vi "PQfetchResultData_experiment.vi"() -> ()   [LabVIEW 2019, in "libpqutility.lvlib"]
uses:
  libpqutility.lvlib
  libpqlv/libpqlv.lvlib
panel:
  in  "conninfo":T1={"host"="localhost", "port"="5432", "client_encoding"="WIN1251", "dbname"="data", "user"="postgres", "password"=""}
  in  "Command":string
  out "DatabaseMesssageCluster":T2
  out "Data":string[][](table)
  out "error out":errorcluster
  in  "error in":errorcluster
  out "PQnTuples":u32
  out "PQnFields":u32
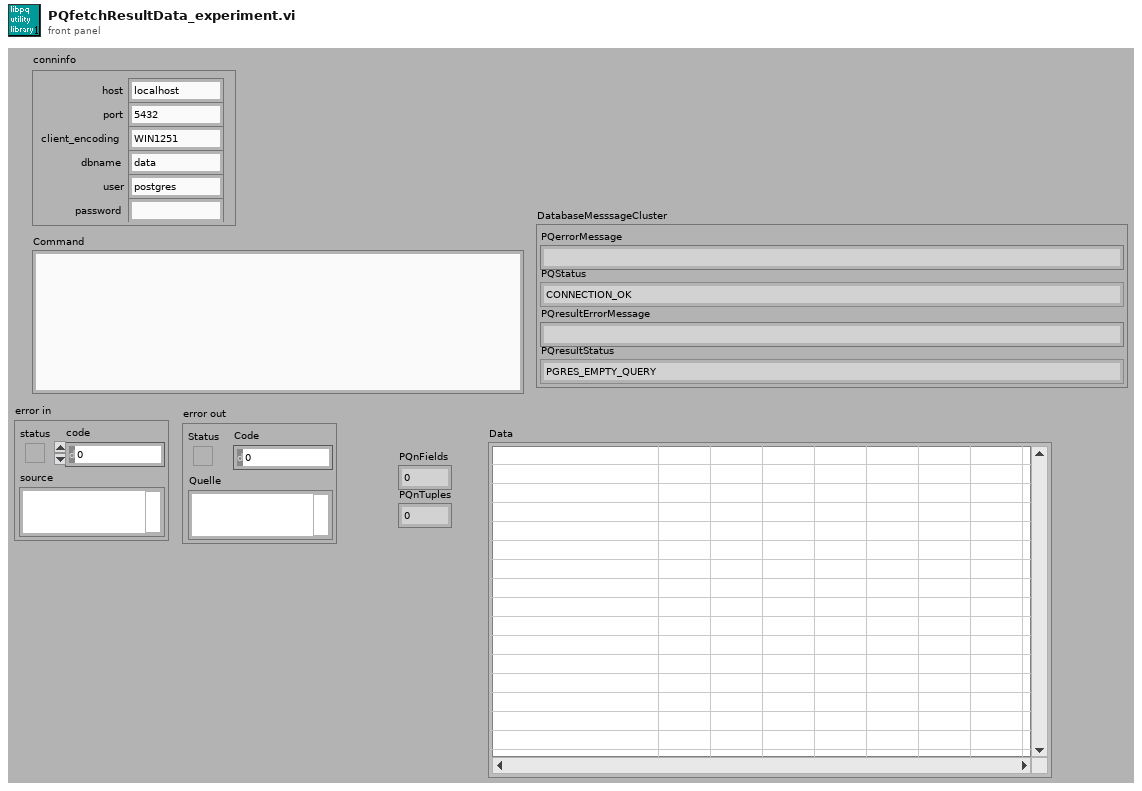
[diagram p1: front panel]
types:
  T1 = cluster{"host":string, "port":string, "client_encoding":string, "dbname":string, "user":string, "password":string}
  T2 = cluster{"PQerrorMessage":string, "PQStatus":enum16{"CONNECTION_OK", "CONNECTION_BAD", "CONNECTION_STARTED", "CONNECTION_MADE", "CONNECTION_AWAITING_RESPONSE", "CONNECTION_AUTH_OK", "CONNECTION_SETENV", "CONNECTION_SSL_STARTUP", "CONNECTION_NEEDED"}, "PQresultErrorMessage":string, "PQresultStatus":enum16{"PGRES_EMPTY_QUERY", "PGRES_COMMAND_OK", "PGRES_TUPLES_OK", "PGRES_COPY_OUT", "PGRES_COPY_IN", "PGRES_BAD_RESPONSE", "PGRES_NONFATAL_ERROR", "PGRES_FATAL_ERROR"}}
  T3 = enum32{"CONNECTION_OK", "CONNECTION_BAD", "CONNECTION_STARTED", "CONNECTION_MADE", "CONNECTION_AWAITING_RESPONSE", "CONNECTION_AUTH_OK", "CONNECTION_SETENV", "CONNECTION_SSL_STARTUP", "CONNECTION_NEEDED"}
  T4 = enum16{"PGRES_EMPTY_QUERY", "PGRES_COMMAND_OK", "PGRES_TUPLES_OK", "PGRES_COPY_OUT", "PGRES_COPY_IN", "PGRES_BAD_RESPONSE", "PGRES_NONFATAL_ERROR", "PGRES_FATAL_ERROR"}
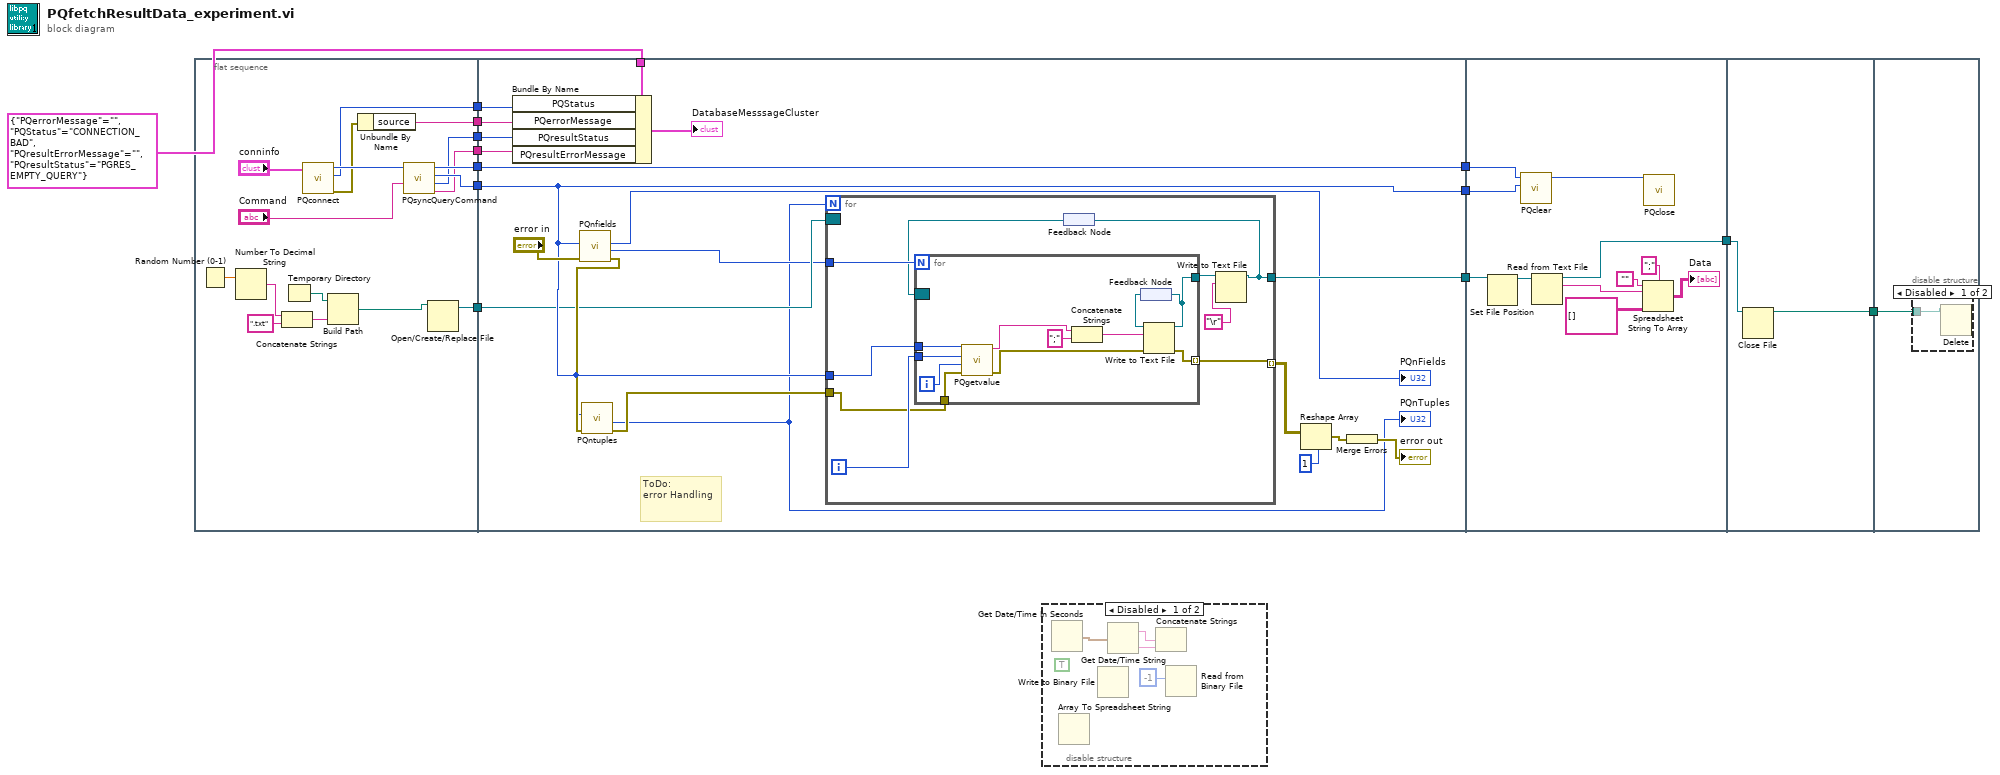
[diagram p0: block diagram]
diagram:
  n1 = flat-sequence {
    tunnel: [w27] -> w10
    tunnel: [w26] -> w8
    tunnel: [w16] -> w6
    tunnel: [w14] -> w5
    tunnel: [w25] -> w4
    tunnel: [w24] -> w3
    tunnel: [w19] -> w1
    tunnel: [w43] -> w13
    tunnel: [w42] -> w11
    tunnel: w10 -> [w42]
    tunnel: [w41] -> w9
    tunnel: w8 -> [w41]
    tunnel: T2 {"PQerrorMessage"="", "PQStatus"=enum."CONNECTION_BAD", "PQresultErrorMessage"="", "PQresultStatus"=enum."PGRES_EMPTY_QUERY"} ("Database Status Message 2") -> [w39]
    tunnel: w6 -> [w38]
    tunnel: w5 -> [w37]
    tunnel: w4 -> [w36]
    tunnel: w3 -> [w35]
    tunnel: w1 -> [w34]
    tunnel: w13 -> [w76]
    tunnel: [w80] -> w12
    tunnel: w11 -> [w78]
    tunnel: w9 -> [w77]
    tunnel: w12 -> [w83]
    tunnel: [w82] -> w2
    tunnel: w2 -> [w84]
    frame #0 {
      n2 = Random Number (0-1)() -> (number: 0 to 1=w29:dbl)
      n3 = Number To Decimal String(number=w29) -> (decimal integer string=w21:string)  [unwired: 1 in]
      n4 = Concatenate Strings(w21, ".txt" ("String")) -> (w22:string)
      n5 = Temporary Directory() -> (w30:path)
      n6 = call "PQconnect.vi"("conninfo"="conninfo") -> ("error out"=w15:errorcluster, "PQStatus"=w16:T3, "conn"=w28:u32)  [unwired: 8 in]
      n7 = Build Path(base path=w30, name or relative path=w22) -> (appended path=w18:path)
      n8 = Unbundle By Name(w15) -> ("source"=w14:string)
      n9 = call "PQsyncQueryCommand.vi"("query"="Command", "conn"=w28) -> ("PQresultErrorMessage"=w24:string, "PQresultStatus"=w25:T4, "PGresult"=w27:u32, "conn out"=w26:u32)  [unwired: 5 in]
      n10 = Open/Create/Replace File(file path (use dialog)=w18) -> (refnum out=w19:refnum<file>)  [unwired: 5 in, 2 out]
    }
    frame #1 {
      # "ToDo:\nerror Handling"
      n11 = Bundle By Name(cluster=w39, "PQStatus"=w38, "PQerrorMessage"=w37, "PQresultStatus"=w36, "PQresultErrorMessage"=w35) -> (→"DatabaseMesssageCluster":T2)
      n12 = call "PQnfields.vi"("error in (no error)"="error in", "res"=w42) -> ("error out"=w49:errorcluster, "PQnFields"=w32:i32, "res out"=→"PQnFields":u32)  [unwired: 7 in]
      n13 = call "PQntuples.vi"("error in (no error)"=w49, "res"=w42) -> ("error out"=w48:errorcluster, "PQnTuples"=w31:i32)  [unwired: 7 in, 1 out]
      "PQnTuples" <- w31
      n14 = for {
        N: w31 -> [_]
        tunnel: w42 -> [w59]
        tunnel: w32 -> [w56]
        tunnel: w48 -> [w57]
        tunnel: [w55] -> w47 mode=indexing
        tunnel: [w53] -> w43
        border: w34 -> [_]
        i -> [w58]
        n15 = feedback #1() -> (w54:refnum<file>)
        n16 = for {
          N: w56 -> [_]
          tunnel: w59 -> [w70]
          tunnel: w58 -> [w68]
          tunnel: w57 -> [w69]
          tunnel: [w65] -> w55 mode=indexing
          tunnel: [w64] -> w52
          border: w54 -> [_]
          i -> [w67]
          n17 = call "PQgetvalue.vi"("error in (no error)"=w69, "column_number"=w67, "row_number"=w68, "res"=w70) -> ("error out"=w66:errorcluster, "field_value"=w60:string)  [unwired: 6 in]
          n18 = Concatenate Strings(w60, ";" ("String")) -> (w62:string)
          n19 = feedback #2() -> (w63:refnum<file>)
          n20 = Write to Text File(file (use dialog)=w63, text=w62, error in=w66) -> (refnum out=w64:refnum<file>, error out=w65:errorcluster)  [unwired: 1 in, 1 out]
          n21 = feedback-in #2(w64) -> ()
        }
        n22 = Write to Text File(file (use dialog)=w52, text="\r") -> (refnum out=w53:refnum<file>)  [unwired: 2 in, 2 out]
        n23 = feedback-in #1(w53) -> ()
      }
      n24 = Reshape Array(w47, 1 ("Dimensionsgröße")) -> (w45:errorcluster[])
      n25 = Merge Errors(w45) -> (→"error out":errorcluster)
    }
    frame #2 {
      n26 = Set File Position(refnum=w76) -> (refnum out=w75:refnum<file>)  [unwired: 3 in, 1 out]
      n27 = call "PQclear.vi"("res"=w78, "conn"=w77) -> ("conn_out"=w79:u32)  [unwired: 8 in, 1 out]
      n28 = Read from Text File(file (use dialog)=w75) -> (refnum out=w80:refnum<file>, text=w81:string)  [unwired: 3 in, 2 out]
      n29 = Spreadsheet String To Array(delimiter (Tab)=";" ("Trennzeichen (Tabulator)"), format string="", spreadsheet string=w81, array type (2D Dbl)=string[][] [] ("Data 2")) -> (array=→"Data":string[][])
      n30 = call "PQclose.vi"("conn"=w79) -> ()  [unwired: 10 in, 1 out]
    }
    frame #3 {
      n31 = Close File(refnum=w83) -> (path=w82:path)  [unwired: 1 in, 1 out]
    }
    frame #4 {
      n32 = disable-structure shown="Disabled" {
        disable-tunnel: w84 -> [w85 _]
        frame Disabled {
          n33 = Delete(path (use dialog)=w85) -> ()  [unwired: 4 in, 3 out]
        }
        frame Enabled {
        }
      }
    }
  }
  n34 = disable-structure shown="Disabled" {
    frame Disabled {
      (unwired) TRUE ("Angabe von Sekunden? (F)")
      n35 = Get Date/Time In Seconds() -> (seconds since 1Jan1904=w87:timestamp)
      n36 = Array To Spreadsheet String() -> ()  [unwired: 3 in, 1 out]
      n37 = Write to Binary File() -> ()  [unwired: 6 in, 3 out]
      n38 = Get Date/Time String(seconds (now)=w87) -> (date string=w88:string, time string=w89:string)  [unwired: 2 in]
      n39 = Concatenate Strings(w88, w89) -> ()  [unwired: 1 in, 1 out]
      n40 = Read from Binary File(10:-1 ("count (1)")) -> ()  [unwired: 5 in, 4 out]
    }
    frame Enabled {
    }
  }
